vi "InitActuators.vi"   [LabVIEW 2020]
uses:
  <vilib>/Rock Robotics/WPI/Solenoid/WPI_SolenoidChannel.ctl
  <vilib>/Rock Robotics/WPI/ThirdParty/Phoenix-LabVIEW/Motor Controller/Controls/CTRE_Phoenix_MotorControl_FeedbackDevice_TalonFX.ctl
  <vilib>/Rock Robotics/WPI/ThirdParty/Phoenix-LabVIEW/Motor Controller/Controls/CTRE_Phoenix_MotorControl_TalonFXInvertType.ctl
  <vilib>/Rock Robotics/WPI/ThirdParty/Phoenix-LabVIEW/Motor Controller/Controls/CTRE_Phoenix_MotorControl_NeutralMode.ctl
  <vilib>/Rock Robotics/WPI/ThirdParty/Phoenix-LabVIEW/Motor Controller/Controls/CTRE_Phoenix_MotorControl_SupplyCurrentLimitConfiguration.ctl
  <vilib>/Rock Robotics/WPI/Solenoid/WPI_SolenoidOpenDouble.vi
  refnums.vi
types:
  T1 = typedef "WPI_SolenoidChannel.ctl" = enum8{"Solenoid 0", "Solenoid 1", "Solenoid 2", "Solenoid 3", "Solenoid 4", "Solenoid 5", "Solenoid 6", "Solenoid 7", "Solenoid 8", "Solenoid 9", "Solenoid 10", "Solenoid 11", "Solenoid 12", "Solenoid 13", "Solenoid 14", "Solenoid 15", "Invalid"}
  T2 = typedef "CTRE_Phoenix_MotorControl_SupplyCurrentLimitConfiguration.ctl" = cluster{"Enable?":bool, "Current Limit":dbl, "Threshold Current":dbl, "Threshold Time":dbl}
  T3 = typedef "CTRE_Phoenix_MotorControl_NeutralMode.ctl" = enum8{"EEPROMSetting", "Override to Coast", "Override to Brake"}
  T4 = typedef "CTRE_Phoenix_MotorControl_TalonFXInvertType.ctl" = enum16{"Counter-Clockwise", "Clockwise"}
  T5 = typedef "CTRE_Phoenix_MotorControl_FeedbackDevice_TalonFX.ctl" = i8
  T6 = typedef "WPI_MotorControlDeviceRef.ctl" = cluster{"DeviceStatus":errorcluster, "Type":T7, "PWM":cluster{"PWM Channel":T8, "DeadBand":T9}, "CAN":cluster{"Device Number":u8, "SetOutput VI Ref":variant, "GetOutput VI Ref":variant, "Enable VI Ref":variant, "Disable VI Ref":variant, "Data":variant}, "Invert":bool, "DIO PWM":cluster{"PWM \"Enable\" Channel":T8, "DIOChannel":T10, "PWM Rate":dbl}}
  T7 = typedef "WPI_MotorControlType.ctl" = enum16{"PWM", "CAN", "DIO PWM"}
  T8 = typedef "FPGA_DIOPWMChannel.ctl" = enum8{"PWM 0", "PWM 1", "PWM 2", "PWM 3", "PWM 4", "PWM 5", "PWM 6", "PWM 7", "PWM 8", "PWM 9", "PWM MXP 0", "PWM MXP 1", "PWM MXP 2", "PWM MXP 3", "PWM MXP 4", "PWM MXP 5", "PWM MXP 6", "PWM MXP 7", "PWM MXP 8", "PWM MXP 9", "Invalid"}
  T9 = typedef "WPI_PWMDeadband.ctl" = cluster{"Name":string, "maxPositivePwm":i32, "minPositivePwm":i32, "centerPwm":i32, "maxNegativePwm":i32, "minNegativePwm":i32, "angularRange":u16}
  T10 = typedef "FPGA_DIOChannel.ctl" = enum8{"DIO 0", "DIO 1", "DIO 2", "DIO 3", "DIO 4", "DIO 5", "DIO 6", "DIO 7", "DIO 8", "DIO 9", "DIO MXP 0", "DIO MXP 1", "DIO MXP 2", "DIO MXP 3", "DIO MXP 4", "DIO MXP 5", "DIO MXP 6", "DIO MXP 7", "DIO MXP 8", "DIO MXP 9", "DIO MXP 10", "DIO MXP 11", "DIO MXP 12", "DIO MXP 13", "DIO MXP 14", "DIO MXP 15", "SPI Port CS1", "SPI Port CS2", "SPI Port CS3", "SPI Port MISO", "SPI Port MOSI", "Invalid"}
  T11 = typedef "WPI_SolenoidDevRef.ctl" = cluster{"DevStatus":errorcluster, "Pneumatics Control Module":u8, "Forward Solenoid Channel":T1, "Reverse Solenoid Channel":T1}
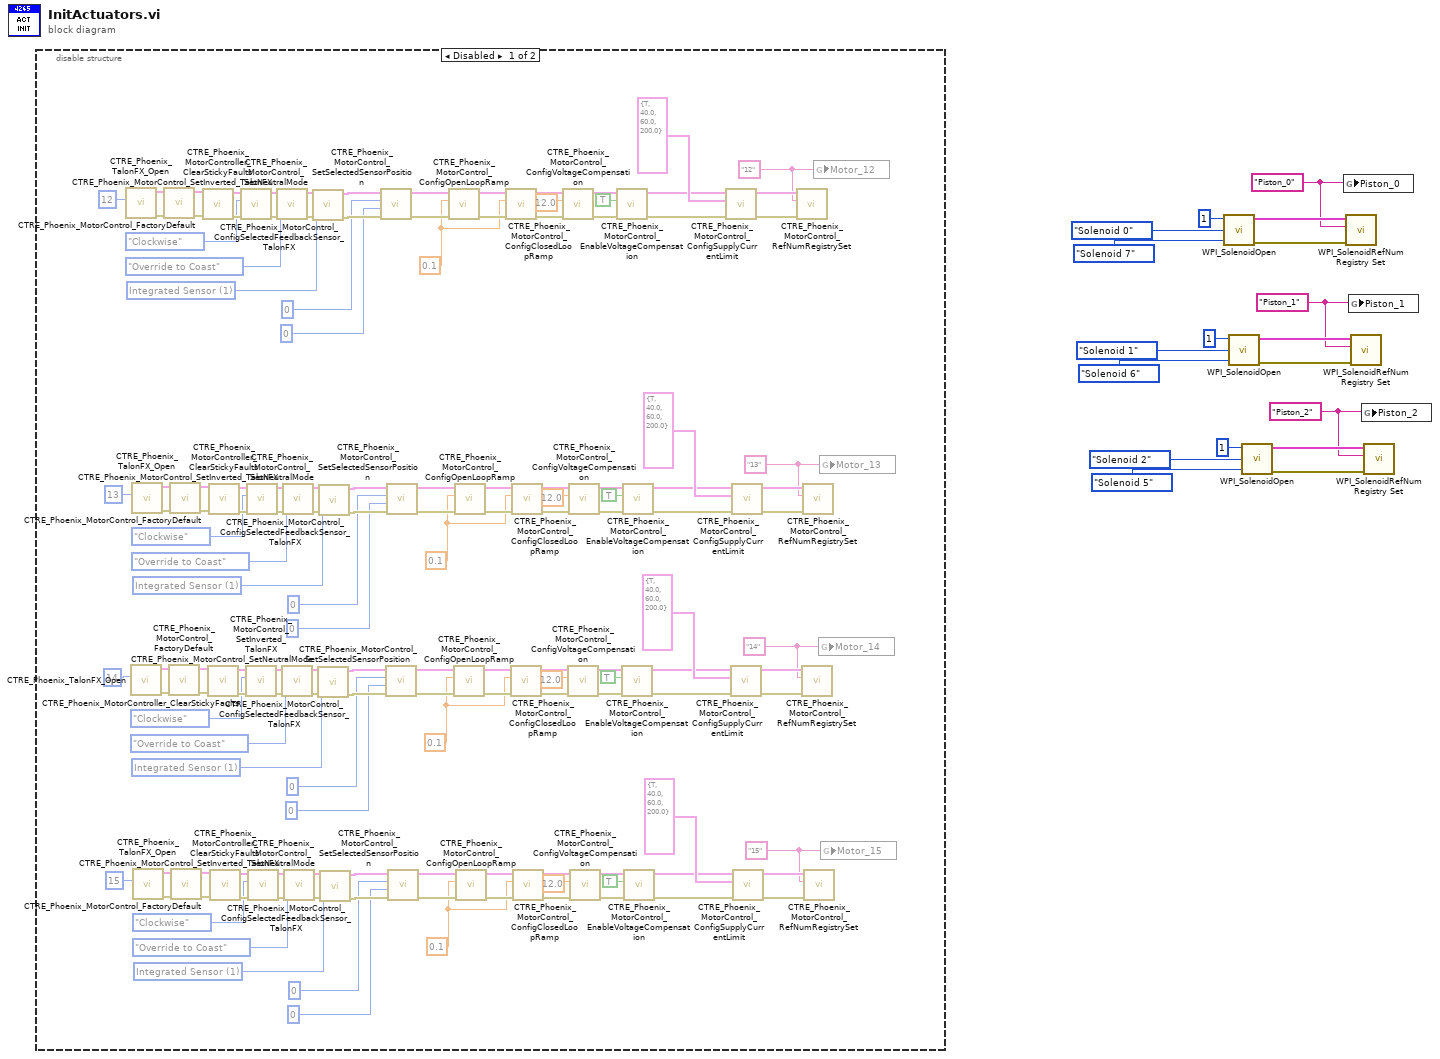
[diagram p0: block diagram]
diagram:
  w1 = "Piston_2" ("refnum name")
  w7 = "Piston_1" ("refnum name")
  w13 = "Piston_0" ("refnum name")
  n1 = disable-structure shown="Disabled" {
    frame Disabled {
      w28 = "12" ("refnum name")
      w31 = 0.1 ("secondsFromNeutralToFull")
      w40 = T5 1 items=["Integrated Sensor"=1, "Sensor Sum (S0 + S1)"=9, "Sensor Difference (D0 - D1)"=10, "Remote Source 0"=11, "Remote Source 1"=12, "None"=14, "Software Emulated"=15] ("Talon FX Feedback Device")
      w63 = "13" ("refnum name")
      w66 = 0.1 ("secondsFromNeutralToFull")
      w75 = T5 1 items=["Integrated Sensor"=1, "Sensor Sum (S0 + S1)"=9, "Sensor Difference (D0 - D1)"=10, "Remote Source 0"=11, "Remote Source 1"=12, "None"=14, "Software Emulated"=15] ("Talon FX Feedback Device")
      w98 = "14" ("refnum name")
      w101 = 0.1 ("secondsFromNeutralToFull")
      w110 = T5 1 items=["Integrated Sensor"=1, "Sensor Sum (S0 + S1)"=9, "Sensor Difference (D0 - D1)"=10, "Remote Source 0"=11, "Remote Source 1"=12, "None"=14, "Software Emulated"=15] ("Talon FX Feedback Device")
      w133 = "15" ("refnum name")
      w136 = 0.1 ("secondsFromNeutralToFull")
      w145 = T5 1 items=["Integrated Sensor"=1, "Sensor Sum (S0 + S1)"=9, "Sensor Difference (D0 - D1)"=10, "Remote Source 0"=11, "Remote Source 1"=12, "None"=14, "Software Emulated"=15] ("Talon FX Feedback Device")
      n2 = call <vilib>:"CTRE_Phoenix_TalonFX_Open.vi"("Device Number"=u8 12) -> ("error out"=w52:errorcluster, "PhoenixMotorControlDevRef"=w51:T6)  [unwired: 9 in]
      n3 = call <vilib>:"CTRE_Phoenix_TalonFX_Open.vi"("Device Number"=u8 14) -> ("error out"=w122:errorcluster, "PhoenixMotorControlDevRef"=w121:T6)  [unwired: 9 in]
      n4 = call <vilib>:"CTRE_Phoenix_TalonFX_Open.vi"("Device Number"=u8 13) -> ("error out"=w87:errorcluster, "PhoenixMotorControlDevRef"=w86:T6)  [unwired: 9 in]
      n5 = call <vilib>:"CTRE_Phoenix_TalonFX_Open.vi"("Device Number"=u8 15) -> ("error out"=w157:errorcluster, "PhoenixMotorControlDevRef"=w156:T6)  [unwired: 9 in]
      n6 = call <vilib>:"CTRE_Phoenix_MotorControl_FactoryDefault.vi"("error in"=w52, "PhoenixMotorControlDevRef"=w51) -> ("error out"=w50:errorcluster, "PhoenixMotorControlDevRef"=w49:T6)  [unwired: 8 in]
      n7 = call <vilib>:"CTRE_Phoenix_MotorControl_FactoryDefault.vi"("error in"=w122, "PhoenixMotorControlDevRef"=w121) -> ("error out"=w120:errorcluster, "PhoenixMotorControlDevRef"=w119:T6)  [unwired: 8 in]
      n8 = call <vilib>:"CTRE_Phoenix_MotorControl_FactoryDefault.vi"("error in"=w87, "PhoenixMotorControlDevRef"=w86) -> ("error out"=w85:errorcluster, "PhoenixMotorControlDevRef"=w84:T6)  [unwired: 8 in]
      n9 = call <vilib>:"CTRE_Phoenix_MotorControl_FactoryDefault.vi"("error in"=w157, "PhoenixMotorControlDevRef"=w156) -> ("error out"=w155:errorcluster, "PhoenixMotorControlDevRef"=w154:T6)  [unwired: 8 in]
      n10 = call <vilib>:"CTRE_Phoenix_MotorController_ClearStickyFaults.vi"("error in"=w50, "PhoenixMotorControlDevRef"=w49) -> ("error out"=w48:errorcluster, "PhoenixMotorControlDevRef"=w47:T6)  [unwired: 8 in]
      n11 = call <vilib>:"CTRE_Phoenix_MotorController_ClearStickyFaults.vi"("error in"=w120, "PhoenixMotorControlDevRef"=w119) -> ("error out"=w118:errorcluster, "PhoenixMotorControlDevRef"=w117:T6)  [unwired: 8 in]
      n12 = call <vilib>:"CTRE_Phoenix_MotorController_ClearStickyFaults.vi"("error in"=w85, "PhoenixMotorControlDevRef"=w84) -> ("error out"=w83:errorcluster, "PhoenixMotorControlDevRef"=w82:T6)  [unwired: 8 in]
      n13 = call <vilib>:"CTRE_Phoenix_MotorController_ClearStickyFaults.vi"("error in"=w155, "PhoenixMotorControlDevRef"=w154) -> ("error out"=w153:errorcluster, "PhoenixMotorControlDevRef"=w152:T6)  [unwired: 8 in]
      n14 = call <vilib>:"CTRE_Phoenix_MotorControl_SetInverted_TalonFX.vi"("error in (no error)"=w48, "Invert Type"=CTRE_Phoenix_MotorControl_TalonFXInvertType."Clockwise", "PhoenixMotorControlDevRef"=w47) -> ("error out"=w45:errorcluster, "PhoenixMotorControlDevRef"=w44:T6)  [unwired: 7 in]
      n15 = call <vilib>:"CTRE_Phoenix_MotorControl_SetInverted_TalonFX.vi"("error in (no error)"=w118, "Invert Type"=CTRE_Phoenix_MotorControl_TalonFXInvertType."Clockwise", "PhoenixMotorControlDevRef"=w117) -> ("error out"=w115:errorcluster, "PhoenixMotorControlDevRef"=w114:T6)  [unwired: 7 in]
      n16 = call <vilib>:"CTRE_Phoenix_MotorControl_SetInverted_TalonFX.vi"("error in (no error)"=w83, "Invert Type"=CTRE_Phoenix_MotorControl_TalonFXInvertType."Clockwise", "PhoenixMotorControlDevRef"=w82) -> ("error out"=w80:errorcluster, "PhoenixMotorControlDevRef"=w79:T6)  [unwired: 7 in]
      n17 = call <vilib>:"CTRE_Phoenix_MotorControl_SetInverted_TalonFX.vi"("error in (no error)"=w153, "Invert Type"=CTRE_Phoenix_MotorControl_TalonFXInvertType."Clockwise", "PhoenixMotorControlDevRef"=w152) -> ("error out"=w150:errorcluster, "PhoenixMotorControlDevRef"=w149:T6)  [unwired: 7 in]
      n18 = call <vilib>:"CTRE_Phoenix_MotorControl_SetNeutralMode.vi"("error in (no error)"=w45, "Motor Control Neutral Mode"=CTRE_Phoenix_MotorControl_NeutralMode."Override to Coast", "PhoenixMotorControlDevRef"=w44) -> ("error out"=w42:errorcluster, "PhoenixMotorControlDevRef"=w41:T6)  [unwired: 7 in]
      n19 = call <vilib>:"CTRE_Phoenix_MotorControl_SetNeutralMode.vi"("error in (no error)"=w115, "Motor Control Neutral Mode"=CTRE_Phoenix_MotorControl_NeutralMode."Override to Coast", "PhoenixMotorControlDevRef"=w114) -> ("error out"=w112:errorcluster, "PhoenixMotorControlDevRef"=w111:T6)  [unwired: 7 in]
      n20 = call <vilib>:"CTRE_Phoenix_MotorControl_SetNeutralMode.vi"("error in (no error)"=w80, "Motor Control Neutral Mode"=CTRE_Phoenix_MotorControl_NeutralMode."Override to Coast", "PhoenixMotorControlDevRef"=w79) -> ("error out"=w77:errorcluster, "PhoenixMotorControlDevRef"=w76:T6)  [unwired: 7 in]
      n21 = call <vilib>:"CTRE_Phoenix_MotorControl_SetNeutralMode.vi"("error in (no error)"=w150, "Motor Control Neutral Mode"=CTRE_Phoenix_MotorControl_NeutralMode."Override to Coast", "PhoenixMotorControlDevRef"=w149) -> ("error out"=w147:errorcluster, "PhoenixMotorControlDevRef"=w146:T6)  [unwired: 7 in]
      n22 = call <vilib>:"CTRE_Phoenix_MotorControl_ConfigSelectedFeedbackSensor_TalonFX.vi"("error in (no error)"=w42, "Talon FX Feedback Device"=w40, "PhoenixMotorControlDevRef"=w41) -> ("error out"=w39:errorcluster, "PhoenixMotorControlDevRef"=w38:T6)  [unwired: 7 in]
      n23 = call <vilib>:"CTRE_Phoenix_MotorControl_ConfigSelectedFeedbackSensor_TalonFX.vi"("error in (no error)"=w112, "Talon FX Feedback Device"=w110, "PhoenixMotorControlDevRef"=w111) -> ("error out"=w109:errorcluster, "PhoenixMotorControlDevRef"=w108:T6)  [unwired: 7 in]
      n24 = call <vilib>:"CTRE_Phoenix_MotorControl_ConfigSelectedFeedbackSensor_TalonFX.vi"("error in (no error)"=w77, "Talon FX Feedback Device"=w75, "PhoenixMotorControlDevRef"=w76) -> ("error out"=w74:errorcluster, "PhoenixMotorControlDevRef"=w73:T6)  [unwired: 7 in]
      n25 = call <vilib>:"CTRE_Phoenix_MotorControl_ConfigSelectedFeedbackSensor_TalonFX.vi"("error in (no error)"=w147, "Talon FX Feedback Device"=w145, "PhoenixMotorControlDevRef"=w146) -> ("error out"=w144:errorcluster, "PhoenixMotorControlDevRef"=w143:T6)  [unwired: 7 in]
      n26 = call <vilib>:"CTRE_Phoenix_MotorControl_SetSelectedSensorPosition.vi"("error in (no error)"=w39, "pidLoopIdx"=u32 0, "New Sensor Position"=0, "PhoenixMotorControlDevRef"=w38) -> ("error out"=w35:errorcluster, "PhoenixMotorControlDevRef"=w34:T6)  [unwired: 6 in]
      n27 = call <vilib>:"CTRE_Phoenix_MotorControl_SetSelectedSensorPosition.vi"("error in (no error)"=w109, "pidLoopIdx"=u32 0, "New Sensor Position"=0, "PhoenixMotorControlDevRef"=w108) -> ("error out"=w105:errorcluster, "PhoenixMotorControlDevRef"=w104:T6)  [unwired: 6 in]
      n28 = call <vilib>:"CTRE_Phoenix_MotorControl_SetSelectedSensorPosition.vi"("error in (no error)"=w74, "pidLoopIdx"=u32 0, "New Sensor Position"=0, "PhoenixMotorControlDevRef"=w73) -> ("error out"=w70:errorcluster, "PhoenixMotorControlDevRef"=w69:T6)  [unwired: 6 in]
      n29 = call <vilib>:"CTRE_Phoenix_MotorControl_SetSelectedSensorPosition.vi"("error in (no error)"=w144, "pidLoopIdx"=u32 0, "New Sensor Position"=0, "PhoenixMotorControlDevRef"=w143) -> ("error out"=w140:errorcluster, "PhoenixMotorControlDevRef"=w139:T6)  [unwired: 6 in]
      n30 = call <vilib>:"CTRE_Phoenix_MotorControl_ConfigOpenLoopRamp.vi"("error in (no error)"=w35, "secondsFromNeutralToFull"=w31, "PhoenixMotorControlDevRef"=w34) -> ("error out"=w33:errorcluster, "PhoenixMotorControlDevRef"=w32:T6)  [unwired: 7 in]
      n31 = call <vilib>:"CTRE_Phoenix_MotorControl_ConfigOpenLoopRamp.vi"("error in (no error)"=w105, "secondsFromNeutralToFull"=w101, "PhoenixMotorControlDevRef"=w104) -> ("error out"=w103:errorcluster, "PhoenixMotorControlDevRef"=w102:T6)  [unwired: 7 in]
      n32 = call <vilib>:"CTRE_Phoenix_MotorControl_ConfigOpenLoopRamp.vi"("error in (no error)"=w70, "secondsFromNeutralToFull"=w66, "PhoenixMotorControlDevRef"=w69) -> ("error out"=w68:errorcluster, "PhoenixMotorControlDevRef"=w67:T6)  [unwired: 7 in]
      n33 = call <vilib>:"CTRE_Phoenix_MotorControl_ConfigOpenLoopRamp.vi"("error in (no error)"=w140, "secondsFromNeutralToFull"=w136, "PhoenixMotorControlDevRef"=w139) -> ("error out"=w138:errorcluster, "PhoenixMotorControlDevRef"=w137:T6)  [unwired: 7 in]
      n34 = call <vilib>:"CTRE_Phoenix_MotorControl_ConfigClosedLoopRamp.vi"("error in (no error)"=w33, "secondsFromNeutralToFull"=w31, "PhoenixMotorControlDevRef"=w32) -> ("error out"=w26:errorcluster, "PhoenixMotorControlDevRef"=w25:T6)  [unwired: 7 in]
      n35 = call <vilib>:"CTRE_Phoenix_MotorControl_ConfigClosedLoopRamp.vi"("error in (no error)"=w103, "secondsFromNeutralToFull"=w101, "PhoenixMotorControlDevRef"=w102) -> ("error out"=w96:errorcluster, "PhoenixMotorControlDevRef"=w95:T6)  [unwired: 7 in]
      n36 = call <vilib>:"CTRE_Phoenix_MotorControl_ConfigClosedLoopRamp.vi"("error in (no error)"=w68, "secondsFromNeutralToFull"=w66, "PhoenixMotorControlDevRef"=w67) -> ("error out"=w61:errorcluster, "PhoenixMotorControlDevRef"=w60:T6)  [unwired: 7 in]
      n37 = call <vilib>:"CTRE_Phoenix_MotorControl_ConfigClosedLoopRamp.vi"("error in (no error)"=w138, "secondsFromNeutralToFull"=w136, "PhoenixMotorControlDevRef"=w137) -> ("error out"=w131:errorcluster, "PhoenixMotorControlDevRef"=w130:T6)  [unwired: 7 in]
      n38 = call <vilib>:"CTRE_Phoenix_MotorControl_ConfigVoltageCompensation.vi"("error in (no error)"=w26, "Saturation Voltage"=12.0, "PhoenixMotorControlDevRef"=w25) -> ("error out"=w23:errorcluster, "PhoenixMotorControlDevRef"=w22:T6)  [unwired: 7 in]
      n39 = call <vilib>:"CTRE_Phoenix_MotorControl_ConfigVoltageCompensation.vi"("error in (no error)"=w96, "Saturation Voltage"=12.0, "PhoenixMotorControlDevRef"=w95) -> ("error out"=w93:errorcluster, "PhoenixMotorControlDevRef"=w92:T6)  [unwired: 7 in]
      n40 = call <vilib>:"CTRE_Phoenix_MotorControl_ConfigVoltageCompensation.vi"("error in (no error)"=w61, "Saturation Voltage"=12.0, "PhoenixMotorControlDevRef"=w60) -> ("error out"=w58:errorcluster, "PhoenixMotorControlDevRef"=w57:T6)  [unwired: 7 in]
      n41 = call <vilib>:"CTRE_Phoenix_MotorControl_ConfigVoltageCompensation.vi"("error in (no error)"=w131, "Saturation Voltage"=12.0, "PhoenixMotorControlDevRef"=w130) -> ("error out"=w128:errorcluster, "PhoenixMotorControlDevRef"=w127:T6)  [unwired: 7 in]
      n42 = call <vilib>:"CTRE_Phoenix_MotorControl_EnableVoltageCompensation.vi"("error in (no error)"=w23, "Enable Voltage Compensation?"=TRUE, "PhoenixMotorControlDevRef"=w22) -> ("error out"=w20:errorcluster, "PhoenixMotorControlDevRef"=w21:T6)  [unwired: 7 in]
      n43 = call <vilib>:"CTRE_Phoenix_MotorControl_EnableVoltageCompensation.vi"("error in (no error)"=w93, "Enable Voltage Compensation?"=TRUE, "PhoenixMotorControlDevRef"=w92) -> ("error out"=w90:errorcluster, "PhoenixMotorControlDevRef"=w91:T6)  [unwired: 7 in]
      n44 = call <vilib>:"CTRE_Phoenix_MotorControl_EnableVoltageCompensation.vi"("error in (no error)"=w58, "Enable Voltage Compensation?"=TRUE, "PhoenixMotorControlDevRef"=w57) -> ("error out"=w55:errorcluster, "PhoenixMotorControlDevRef"=w56:T6)  [unwired: 7 in]
      n45 = call <vilib>:"CTRE_Phoenix_MotorControl_EnableVoltageCompensation.vi"("error in (no error)"=w128, "Enable Voltage Compensation?"=TRUE, "PhoenixMotorControlDevRef"=w127) -> ("error out"=w125:errorcluster, "PhoenixMotorControlDevRef"=w126:T6)  [unwired: 7 in]
      n46 = call <vilib>:"CTRE_Phoenix_MotorControl_ConfigSupplyCurrentLimit.vi"("error in (no error)"=w20, "Supply Current Limit Configuration"=T2 {"Enable?"=TRUE, "Current Limit"=40.0, "Threshold Current"=60.0, "Threshold Time"=200.0}, "PhoenixMotorControlDevRef"=w21) -> ("error out"=w30:errorcluster, "PhoenixMotorControlDevRef"=w29:T6)  [unwired: 7 in]
      n47 = call <vilib>:"CTRE_Phoenix_MotorControl_ConfigSupplyCurrentLimit.vi"("error in (no error)"=w90, "Supply Current Limit Configuration"=T2 {"Enable?"=TRUE, "Current Limit"=40.0, "Threshold Current"=60.0, "Threshold Time"=200.0}, "PhoenixMotorControlDevRef"=w91) -> ("error out"=w100:errorcluster, "PhoenixMotorControlDevRef"=w99:T6)  [unwired: 7 in]
      n48 = call <vilib>:"CTRE_Phoenix_MotorControl_ConfigSupplyCurrentLimit.vi"("error in (no error)"=w55, "Supply Current Limit Configuration"=T2 {"Enable?"=TRUE, "Current Limit"=40.0, "Threshold Current"=60.0, "Threshold Time"=200.0}, "PhoenixMotorControlDevRef"=w56) -> ("error out"=w65:errorcluster, "PhoenixMotorControlDevRef"=w64:T6)  [unwired: 7 in]
      n49 = call <vilib>:"CTRE_Phoenix_MotorControl_ConfigSupplyCurrentLimit.vi"("error in (no error)"=w125, "Supply Current Limit Configuration"=T2 {"Enable?"=TRUE, "Current Limit"=40.0, "Threshold Current"=60.0, "Threshold Time"=200.0}, "PhoenixMotorControlDevRef"=w126) -> ("error out"=w135:errorcluster, "PhoenixMotorControlDevRef"=w134:T6)  [unwired: 7 in]
      n50 = call <vilib>:"CTRE_Phoenix_MotorControl_RefNumRegistrySet.vi"("error in (no error)"=w30, "refnum name"=w28, "PhoenixMotorControlDevRef"=w29) -> ()  [unwired: 7 in, 2 out]
      n51 = call <vilib>:"CTRE_Phoenix_MotorControl_RefNumRegistrySet.vi"("error in (no error)"=w100, "refnum name"=w98, "PhoenixMotorControlDevRef"=w99) -> ()  [unwired: 7 in, 2 out]
      n52 = call <vilib>:"CTRE_Phoenix_MotorControl_RefNumRegistrySet.vi"("error in (no error)"=w65, "refnum name"=w63, "PhoenixMotorControlDevRef"=w64) -> ()  [unwired: 7 in, 2 out]
      n53 = call <vilib>:"CTRE_Phoenix_MotorControl_RefNumRegistrySet.vi"("error in (no error)"=w135, "refnum name"=w133, "PhoenixMotorControlDevRef"=w134) -> ()  [unwired: 7 in, 2 out]
      n54 = global write "refnums.vi" "Motor_12"(w28) -> ()
      n55 = global write "refnums.vi" "Motor_14"(w98) -> ()
      n56 = global write "refnums.vi" "Motor_13"(w63) -> ()
      n57 = global write "refnums.vi" "Motor_15"(w133) -> ()
    }
    frame Enabled {
    }
  }
  n58 = call-poly <vilib>:"WPI_SolenoidOpen.vi"("Reverse Solenoid Channel"=WPI_SolenoidChannel."Solenoid 7", "Forward Solenoid Channel"=WPI_SolenoidChannel."Solenoid 0", "Pneumatics Device (def)"=u8 1) -> ("error out"=w15:errorcluster, "SolenoidDevRef"=w14:T11)  [unwired: 7 in]
  n59 = call-poly <vilib>:"WPI_SolenoidOpen.vi"("Reverse Solenoid Channel"=WPI_SolenoidChannel."Solenoid 6", "Forward Solenoid Channel"=WPI_SolenoidChannel."Solenoid 1", "Pneumatics Device (def)"=u8 1) -> ("error out"=w9:errorcluster, "SolenoidDevRef"=w8:T11)  [unwired: 7 in]
  n60 = call-poly <vilib>:"WPI_SolenoidOpen.vi"("Reverse Solenoid Channel"=WPI_SolenoidChannel."Solenoid 5", "Forward Solenoid Channel"=WPI_SolenoidChannel."Solenoid 2", "Pneumatics Device (def)"=u8 1) -> ("error out"=w3:errorcluster, "SolenoidDevRef"=w2:T11)  [unwired: 7 in]
  n61 = global write "refnums.vi" "Piston_0"(w13) -> ()
  n62 = call <vilib>:"WPI_SolenoidRefNum Registry Set.vi"("error in (no error)"=w15, "refnum name"=w13, "SolenoidDevRef"=w14) -> ()  [unwired: 7 in, 2 out]
  n63 = global write "refnums.vi" "Piston_1"(w7) -> ()
  n64 = call <vilib>:"WPI_SolenoidRefNum Registry Set.vi"("error in (no error)"=w9, "refnum name"=w7, "SolenoidDevRef"=w8) -> ()  [unwired: 7 in, 2 out]
  n65 = global write "refnums.vi" "Piston_2"(w1) -> ()
  n66 = call <vilib>:"WPI_SolenoidRefNum Registry Set.vi"("error in (no error)"=w3, "refnum name"=w1, "SolenoidDevRef"=w2) -> ()  [unwired: 7 in, 2 out]
